vi "Step_1_Ans_AR.vi"   [LabVIEW 2012]
types:
  T1 = typedef "BotSpeak_Control.ctl" = cluster{"Address":string, "Reply EOF":string, "Hardware":string, "Retries":i8, "Timeout":i32}
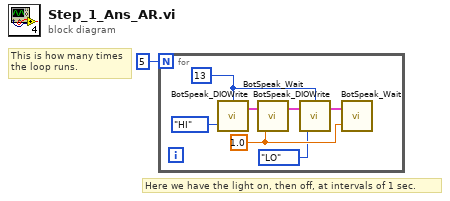
[diagram p0: block diagram]
diagram:
  # "Here we have the light on, then off, at intervals of 1 sec."
  # "This is how many times the loop runs."
  n1 = for {
    N: 5 -> [_]
    w4 = 1.0 ("Wait (sec)")
    w5 = u32 13 ("DIO Line")
    n2 = call <userlib>:"BotSpeak_DIOWrite.vi"("State"=enum32{"LO", "HI"}."HI", "DIO Line"=w5) -> ("Bot Settings"=w8:T1)  [unwired: 1 in, 1 out]
    n3 = call <userlib>:"BotSpeak_Wait.vi"("Wait (sec)"=w4, "Bot Settings"=w8) -> ("Bot Settings"=w7:T1)  [unwired: 1 in]
    n4 = call <userlib>:"BotSpeak_DIOWrite.vi"("State"=enum32{"LO", "HI"}."LO", "Bot Settings"=w7, "DIO Line"=w5) -> ("Bot Settings"=w6:T1)  [unwired: 1 out]
    n5 = call <userlib>:"BotSpeak_Wait.vi"("Wait (sec)"=w4, "Bot Settings"=w6) -> ()  [unwired: 1 in, 1 out]
  }
